vi "Read.vi"(8 "error in (no error)":errorcluster, 11 "CryoCoolerAVC in":refnum<class "CryoCoolerAVC.lvclass">) -> (0 "error out":errorcluster, 2 "Data":dbl[](array[numeric]), 3 "CryoCoolerAVC out":refnum<class "CryoCoolerAVC.lvclass">)   [LabVIEW 2024, in "CryoCoolerAVC.lvclass"]
uses:
  CryoCoolerAVC.lvclass
  CryoCoolerAVC.lvclass/CryoCoolerAVC.ctl
  Cryo Cooler.lvclass
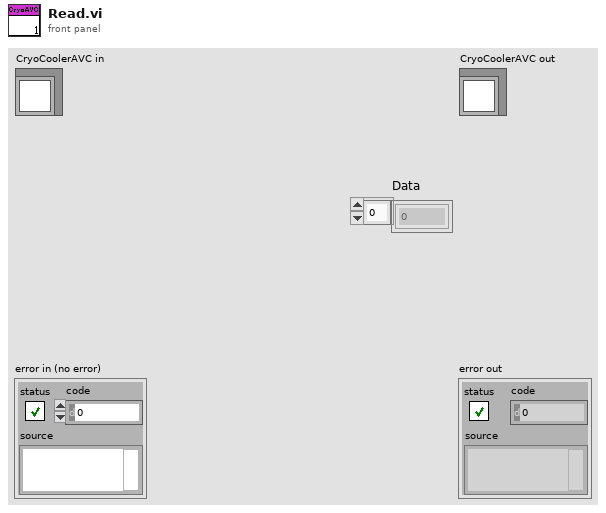
[diagram p1: front panel]
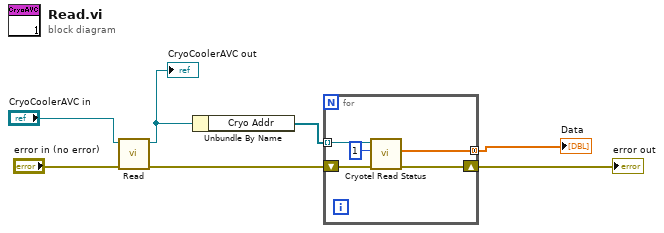
[diagram p0: block diagram]
diagram:
  n1 = call-parent "Read.vi"("error in (no error)"="error in (no error)", "Cryo Cooler in"="CryoCoolerAVC in") -> ("error out"=w5:errorcluster, "Cryo Cooler out"=w4:refnum<class "CryoCoolerAVC.lvclass">)  [unwired: 7 in, 1 out]
  "CryoCoolerAVC out" <- w4
  n2 = Unbundle By Name(w4) -> ("Cryo Addr"=w3:refnum<visa-resource-name>[])
  n3 = for {
    tunnel: w3 -> [w11] mode=indexing
    tunnel: [w8] -> w1 mode=concatenating
    shift-right: [w9] -> w2
    shift-left: w5 -> [w12]
    n4 = call "Cryotel Read Status.vi"("error in"=w12, "Number of reads"=1, "VISA Resource (write)"=w11) -> ("error out"=w9:errorcluster, "Data"=w8:dbl[])  [unwired: 6 in, 1 out]
  }
  "error out" <- w2
  "Data" <- w1
